vi "readEnvVar.vi"(11 "command line":string) -> (3 "standard output":string)   [LabVIEW 2016]
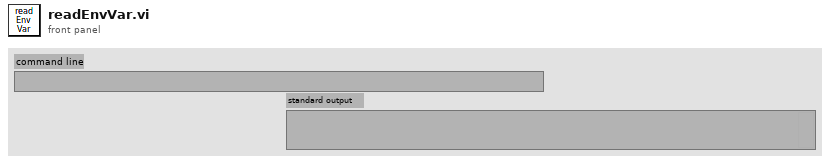
[diagram p1: front panel]
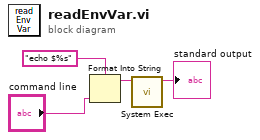
[diagram p0: block diagram]
diagram:
  n1 = Format Into String(format string="echo $%s", "command line") -> (resulting string=w1:string)  [unwired: 2 in, 1 out]
  n2 = call <vilib>:"System Exec.vi"("command line"=w1) -> ("standard output"=→"standard output":string)  [unwired: 7 in, 3 out]
